vi "Invoke IL Action.vi"(8 "error in (no error)":errorcluster, 11 "Interlock in":refnum<class "Interlock.lvclass">) -> (0 "error out":errorcluster, 3 "Interlock out":refnum<class "Interlock.lvclass">)   [LabVIEW 2015, in "Interlocks.lvlib" / "Interlock.lvclass"]
uses:
  Interlock.lvclass
  Interlock.lvclass/Interlock.ctl
  IL Action/IL Action.lvclass/IL Action.ctl
  <vilib>/ActorFramework/Message Enqueuer/Message Enqueuer.lvclass/Message Enqueuer.ctl
  <vilib>/ActorFramework/Message Priority Queue/Priority Enqueue.vi
  IL Action/IL Action.lvclass
  <vilib>/ActorFramework/Message Enqueuer/Message Enqueuer.lvclass
panel:
  out "Name":string
  out "error out 2":errorcluster
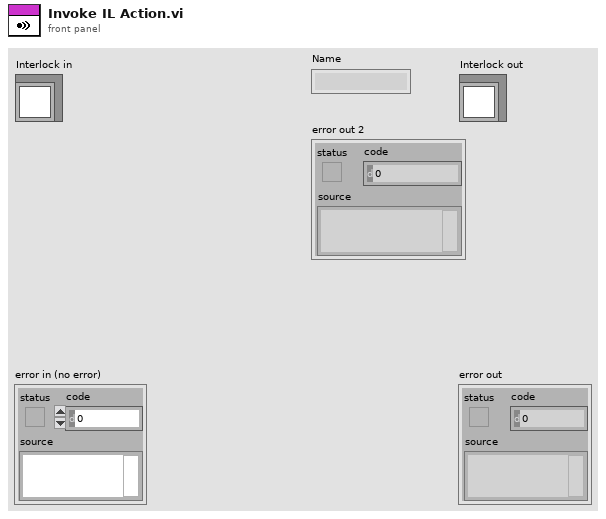
[diagram p1: front panel]
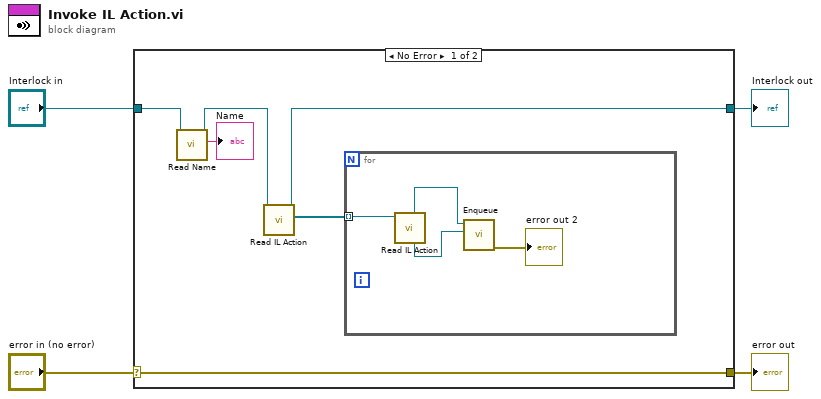
[diagram p0: block diagram]
diagram:
  n1 = case shown="No Error" "error in (no error)" {
    selector: "error in (no error)" -> [w10 w16]
    tunnel: [w10 w16] -> w3
    tunnel: [w8 w15] -> w1
    tunnel: "Interlock in" -> [w7 w15]
    frame No Error {
      n2 = call "Read Name.vi"("Interlock in"=w7) -> ("Name"=→"Name":string, "Interlock out"=w6:refnum<class "Interlock.lvclass">)  [unwired: 9 in]
      n3 = call "Read IL Action.vi"("Interlock in"=w6) -> ("IL Action"=w9:refnum<class "IL Action.lvclass">[], "Interlock out"=w8:refnum<class "Interlock.lvclass">)  [unwired: 9 in]
      n4 = for {
        tunnel: w9 -> [w14] mode=indexing
        n5 = call "Read IL Action.vi"("IL Action in"=w14) -> ("Actor Framework:Message"=w12:refnum<class "Message.lvclass">, "Action Destination"=w13:refnum<class "Message Enqueuer.lvclass">)  [unwired: 7 in, 2 out]
        n6 = call <vilib>:"Enqueue.vi"("Message"=w12, "Message Enqueuer in"=w13) -> ("error out"=→"error out 2":errorcluster)  [unwired: 8 in, 1 out]
      }
    }
    frame Error {
    }
  }
  "error out" <- w3
  "Interlock out" <- w1
